vi "Petrify Code.vi"(6 "State In":T7, 7 "Terms":T2, 8 "error in (no error)":errorcluster, 9 "XRef":T6, 10 "Diagram":T1, 11 "VI in":refnum<vi>) -> (0 "error out":errorcluster)   [LabVIEW 2012, in "OpenG FilterArray.xnode"]
uses:
  OpenG FilterArray.xnode
  State.ctl
  <vilib>/XNodeSupport/XNodeXNodeRef.ctl
  <vilib>/XNodeSupport/XNodeTermIDPairs.ctl
  <vilib>/XNodeSupport/XNodeTermIDPair.ctl
  <vilib>/XNodeSupport/XNodeTermRef.ctl
  <vilib>/XNodeSupport/XNodeString.ctl
  <vilib>/XNodeSupport/XNodeTopLevelDiagramRef.ctl
  <vilib>/Utility/miscctls.llb/LVPositionTypeDef.ctl
  <userlib>/_LAVAcr/Scripting Tools/Scripting Tools.lvlib
  <vilib>/XNodeSupport/NI_XNodeSupport.lvlib
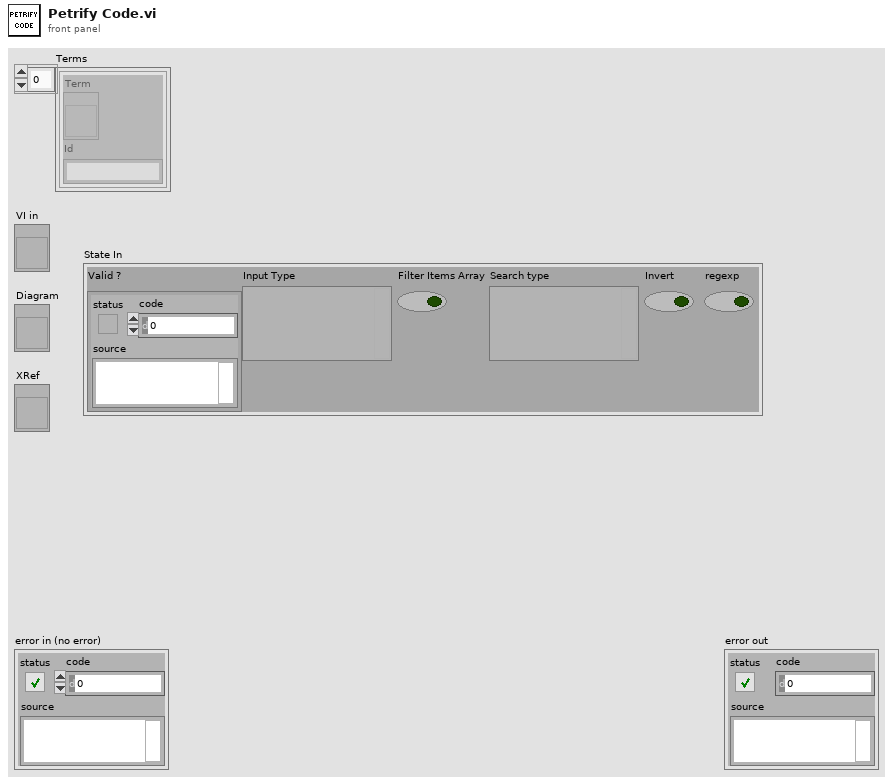
[diagram p1: front panel]
types:
  T1 = typedef "NI_XNodeSupport.lvlib/XNodeTopLevelDiagramRef.ctl" = refnum<vi>
  T2 = typedef "NI_XNodeSupport.lvlib/XNodeTermIDPairs.ctl" = T3[]
  T3 = typedef "NI_XNodeSupport.lvlib/XNodeTermIDPair.ctl" = cluster{"Term":T4, "Id":T5}
  T4 = typedef "NI_XNodeSupport.lvlib/XNodeTermRef.ctl" = refnum<vi>
  T5 = typedef "NI_XNodeSupport.lvlib/XNodeString.ctl" = string
  T6 = typedef "NI_XNodeSupport.lvlib/XNodeXNodeRef.ctl" = refnum<vi>
  T7 = typedef "OpenG FilterArray.xnode/State.ctl" = cluster{"Valid ?":errorcluster, "Input Type":variant, "Filter Items Array":bool, "Search type":variant, "Invert":bool, "regexp":bool}
  T8 = cluster{"left":i16, "top":i16, "right":i16, "bottom":i16}
  T9 = typedef "LVPositionTypeDef.ctl" = cluster{"Left":i32, "Top":i32}
  T10 = typedef "NI_XNodeSupport.lvlib/XNodeInt.ctl" = i32
  T11 = cluster{"Alignment":enum32{"Left", "Right", "Hybrid", "Center", "Gravity"}, "Rules":enum32{"Strict", "Allow Wires Under Labels", "Allow Wires Under Lead Nodes", "Allow Wires Under Wide Blocks"}, "Max Heuristic Iterations":u32, "Max Simplex Iterations":u32, "Block Padding":cluster{"Horizontal":i32, "Vertical":i32}, "Wire Padding":cluster{"Horizontal":i32, "Vertical":i32}, "Auto-Tune by Topology":bool, "Fine-Tune Y Positions":bool, "Align All Controls on Left":bool, "Align All Indicators on Right":bool, "Use Array Dimension Heuristics":bool}
  T12 = typedef "imagedata.ctl" = cluster{"image type":i32, "image depth":i32, "image":u8[], "mask":u8[], "colors":u32[], "Rectangle":cluster{"left":i16, "top":i16, "right":i16, "bottom":i16}}
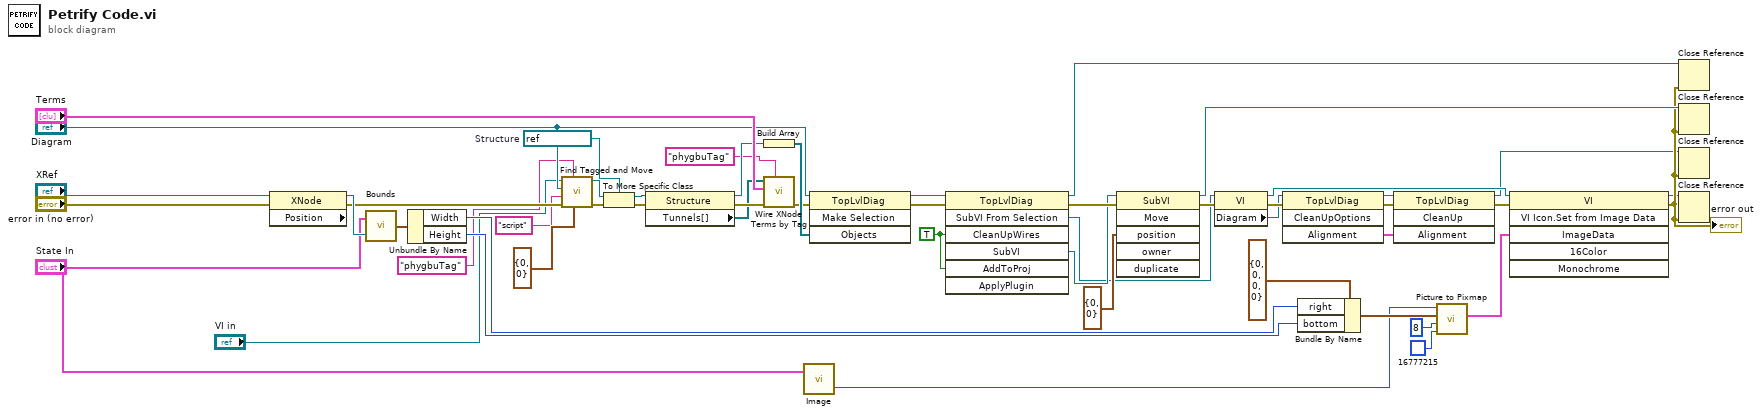
[diagram p0: block diagram]
diagram:
  w25 = TRUE ("Clean Up Wires")
  w2 = refnum<vi> refnum  # Structure
  n1 = property class="XNode" props=["Position"](reference="XRef", error in="error in (no error)") -> (reference out=w24:T6, error out=w22:errorcluster)  [unwired: 1 out]
  n2 = call "Bounds.vi"("XRef"=w24, "State In"="State In") -> ("Bounds"=w47:cluster{"Width":T10, "Height":T10})
  n3 = Unbundle By Name(w47) -> ("Width"=w48:T10, "Height"=w49:T10)
  n4 = call <userlib>:"Find Tagged and Move.vi"("position"=T9 {"Left"=0, "Top"=0}, "TagName"="phygbuTag", "error in"=w22, "TagValue"="script", "Destination Diagram"="Diagram", "VI Refnum"="VI in") -> ("error out"=w8:errorcluster, "Moved Tagged object"=w7:refnum<vi>)  [unwired: 4 out]
  n5 = To More Specific Class(target class=w2, reference=w7, error in=w8) -> (specific class reference=w1:refnum<vi>, error out=w9:errorcluster)
  n6 = property class="Structure"(reference=w1, error in=w9) -> (reference out=w15:refnum<vi>, error out=w10:errorcluster, "Tunnels[]"=w3:refnum<vi>[])
  n7 = Build Array(w15) -> (w16:refnum<vi>[])
  n8 = call <userlib>:"Wire XNode Terms by Tag.vi"("TagName"="phygbuTag", "error in (no error)"=w10, "Term Refs"="Terms", "Source References"=w3) -> ("error out"=w14:errorcluster)  [unwired: 7 out]
  n9 = call "Image.vi"("State In"="State In") -> ("Image"=w42:picture)  [unwired: 2 in]
  n10 = invoke class="TopLvlDiag" method="Make Selection"(reference="Diagram", error in=w14, "Objects"=w16) -> (reference out=w18:T1, error out=w17:errorcluster)  [unwired: 1 in, 2 out]
  n11 = invoke class="TopLvlDiag" method="SubVI From Selection"(reference=w18, error in=w17, "CleanUpWires"=w25, "AddToProj"=w25) -> (reference out=w34:T1, error out=w37:errorcluster, "SubVIFromSelection"=w26:refnum<vi>, "SubVI"=w36:refnum<vi>)  [unwired: 3 in, 3 out]
  n12 = invoke class="SubVI" method="Move"(reference=w36, error in=w37, "position"=T9 {"Left"=0, "Top"=0}) -> (reference out=w39:refnum<vi>, error out=w38:errorcluster)  [unwired: 3 in, 4 out]
  n13 = property class="VI"(reference=w26, error in=w38) -> (reference out=w40:refnum<vi>, error out=w30:errorcluster, "Diagram"=w27:refnum<vi>)
  n14 = invoke class="TopLvlDiag" method="CleanUpOptions"(reference=w27, error in=w30) -> (reference out=w28:refnum<vi>, error out=w31:errorcluster, "Alignment"=w29:T11)  [unwired: 2 in, 1 out]
  n15 = Bundle By Name(cluster=T8 {"left"=0, "top"=0, "right"=0, "bottom"=0} ("rect"), "right"=w48, "bottom"=w49) -> (w46:T8)
  n16 = invoke class="TopLvlDiag" method="CleanUp"(reference=w28, error in=w31, "Alignment"=w29) -> (reference out=w33:refnum<vi>, error out=w50:errorcluster)  [unwired: 1 in, 2 out]
  n17 = call <vilib>:"Picture to Pixmap.vi"("Background Color"=u32 16777215, "depth"=8, "rect"=w46, "picture"=w42) -> ("image data"=w51:T12)  [unwired: 6 in, 1 out]
  n18 = invoke class="VI" method="VI Icon.Set from Image Data"(reference=w40, error in=w50, "ImageData"=w51) -> (reference out=w32:refnum<vi>, error out=w35:errorcluster)  [unwired: 3 in, 4 out]
  "error out" <- w35
  n19 = Close Reference(reference=w34, error in (no error)=w35) -> ()  [unwired: 1 out]
  n20 = Close Reference(reference=w39, error in (no error)=w35) -> ()  [unwired: 1 out]
  n21 = Close Reference(reference=w33, error in (no error)=w35) -> ()  [unwired: 1 out]
  n22 = Close Reference(reference=w32, error in (no error)=w35) -> ()  [unwired: 1 out]
